vi "Write VariableGroups.vi"(8 "error in (no error)":errorcluster, 10 "VariableGroups":refnum<class "VariableGroup.lvclass">[](array[class]), 11 "VariableManager in":refnum<class "VariableManager.lvclass">) -> (0 "error out":errorcluster, 3 "VariableManager out":refnum<class "VariableManager.lvclass">)   [LabVIEW 2013, in "VariableManager.lvclass"]
uses:
  VariableManager.lvclass
  VariableGroup/VariableGroup.lvclass
  VariableManager.lvclass/VariableManager.ctl
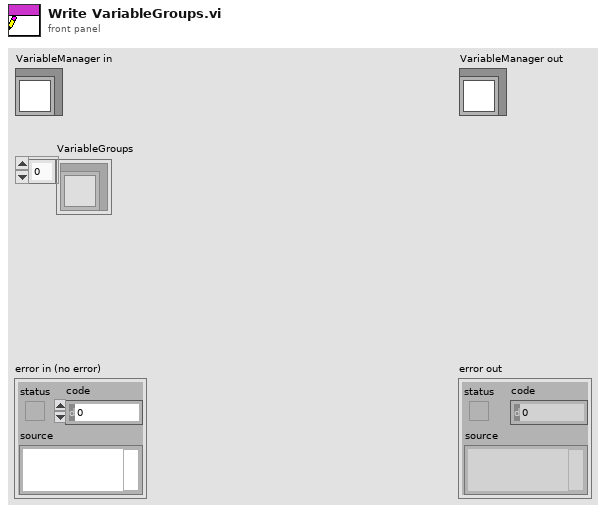
[diagram p1: front panel]
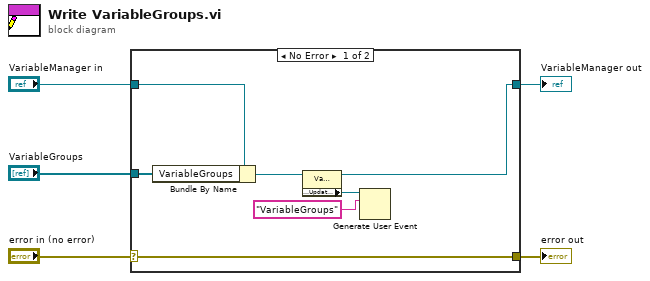
[diagram p0: block diagram]
diagram:
  n1 = case shown="No Error" "error in (no error)" {
    selector: "error in (no error)" -> [w12 w13]
    tunnel: [w12 w13] -> w4
    tunnel: [w6 w14] -> w2
    tunnel: "VariableManager in" -> [w11 w14]
    tunnel: "VariableGroups" -> [w10 _]
    frame No Error {
      n2 = Bundle By Name(cluster=w11, "VariableGroups"=w10) -> (w7:refnum<class "VariableManager.lvclass">)
      n3 = property class="VariableManager.lvclass"(reference=w7) -> (reference out=w6:refnum<class "VariableManager.lvclass">, "Accessors:UpdateEvent"=w9:refnum<user-event>)  [unwired: 1 in, 1 out]
      n4 = Generate User Event(user event=w9, event data cluster="VariableGroups") -> ()  [unwired: 2 in, 2 out]
    }
    frame Error {
    }
  }
  "error out" <- w4
  "VariableManager out" <- w2
